vi "Turret_Manual_Aim.vi"   [LabVIEW 2011]
uses:
  StateMachineType.ctl
  Robot Global Data.vi
types:
  T1 = typedef "StateMachineType.ctl" = enum16{"Init", "Idle", "Start", "Do", "Stop"}
  T2 = typedef "WPI_MotorControlDeviceRef.ctl" = cluster{"DeviceStatus":errorcluster, "Type":enum16{"PWM", "CAN"}, "PWM":cluster{"Digital Module":T3, "PWM Channel":T4, "DeadBand":T5}, "CAN":cluster{"Device Number":u8, "Control Mode":T6, "Semaphore":T7, "Max Vout":dbl}, "Invert":bool, "TransformRef":T8, "InvTransformRef":T8}
  T3 = typedef "FPGA_TypedefDigitalModule.ctl" = enum16{"Digital Module 1", "Digital Module 2"}
  T4 = typedef "FPGA_DIOPWMChannel.ctl" = enum8{"PWM 1", "PWM 2", "PWM 3", "PWM 4", "PWM 5", "PWM 6", "PWM 7", "PWM 8", "PWM 9", "PWM 10", "Invalid"}
  T5 = typedef "WPI_PWMDeadband.ctl" = cluster{"Name":string, "maxPositivePwm":i32, "minPositivePwm":i32, "centerPwm":i32, "maxNegativePwm":i32, "minNegativePwm":i32, "angularRange":u16}
  T6 = typedef "WPI_CANJaguar_ControlMode.ctl" = enum8{"Percent VBus", "Current", "Speed", "Position", "Voltage"}
  T7 = typedef "Semaphore RefNum" = refnum<k1>
  T8 = typedef "WPI_PWMTransform_ConPane.ctl" = refnum<vi>
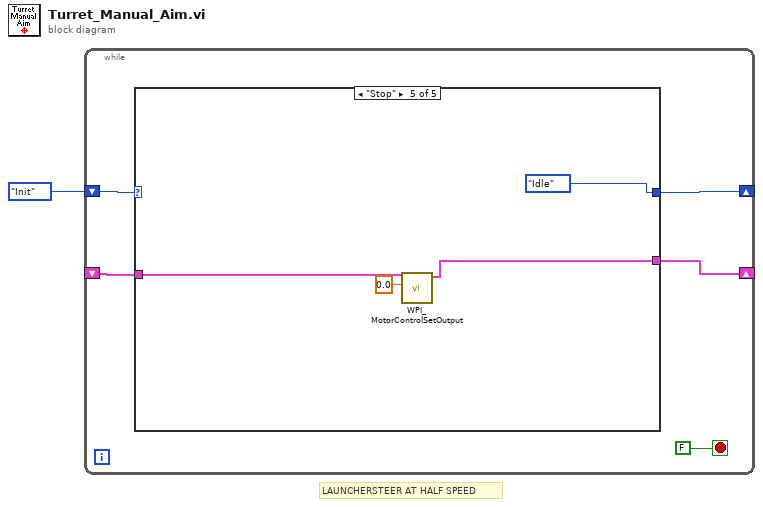
[diagram p0: block diagram]
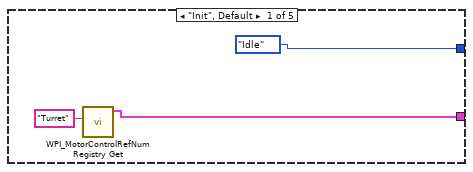
[diagram p2: hidden frame]
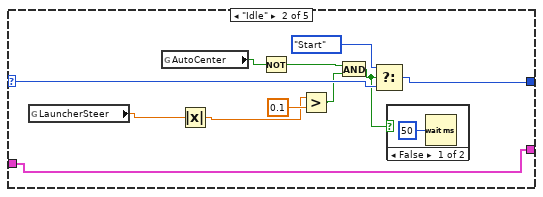
[diagram p3: hidden frame]
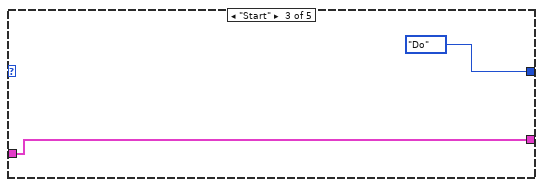
[diagram p5: hidden frame]
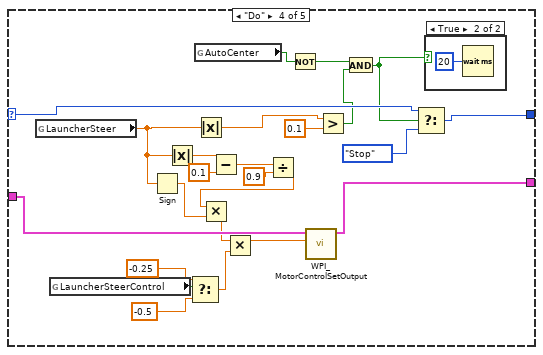
[diagram p6: hidden frame]
diagram:
  # "LAUNCHERSTEER AT HALF SPEED"
  n1 = while {
    shift-right: [w4] -> _
    shift-left: StateMachineType."Init" -> [w5]
    shift-right: [w3] -> _
    shift-left: _ -> [w2]
    stop <- FALSE stop-if-true
    n2 = case shown="\"Stop\"" w5 {
      selector: w5 -> [_ w19 _ w44 _]
      tunnel: [StateMachineType."Idle" ("Enum") w18 StateMachineType."Do" ("Enum") w45 StateMachineType."Idle" ("Enum")] -> w4
      tunnel: [w7 w16 w23 w41 w50] -> w3
      tunnel: w2 -> [_ w16 w23 w42 w51]
      frame "Init", Default {
        n3 = call <vilib>:"WPI_MotorControlRefNum Registry Get.vi"("refnum name"="Turret") -> ("MotorControlDevRef"=w7:T2)  [unwired: 9 in, 1 out]
      }
      frame "Idle" {
        n4 = global read "Robot Global Data.vi" "LauncherSteer"() -> (w15:dbl)
        n5 = global read "Robot Global Data.vi" "AutoCenter"() -> (w13:bool)
        n6 = Absolute Value(x=w15) -> (abs(x)=w14:dbl)
        n7 = Not(x=w13) -> (.not. x?=w11:bool)
        n8 = Greater?(x=w14, y=0.1) -> (0:w12:bool)
        n9 = And(x=w11, y=w12) -> (x .and. y?=w10:bool)
        n10 = Select(t=StateMachineType."Start" ("Enum"), s=w10, f=w19) -> (s? t:f=w18:T1)
        n11 = case shown="False" w10 {
          frame False {
            n12 = Wait (ms)(milliseconds to wait=u32 50) -> ()  [unwired: 1 out]
          }
          frame True {
          }
        }
      }
      frame "Start" {
      }
      frame "Do" {
        n13 = global read "Robot Global Data.vi" "LauncherSteer"() -> (w27:dbl)
        n14 = global read "Robot Global Data.vi" "LauncherSteerControl"() -> (w35:bool)
        n15 = Sign(1:w27) -> (0:w26:dbl)
        n16 = Absolute Value(x=w27) -> (abs(x)=w31:dbl)
        n17 = Select(t=-0.25 ("y"), s=w35, f=-0.5 ("y")) -> (s? t:f=w32:dbl)
        n18 = global read "Robot Global Data.vi" "AutoCenter"() -> (w39:bool)
        n19 = Absolute Value(x=w27) -> (abs(x)=w43:dbl)
        n20 = Subtract(x=w31, y=0.1) -> (x-y=w30:dbl)
        n21 = Divide(x=w30, y=0.9) -> (x/y=w25:dbl)
        n22 = Multiply(x=w25, y=w26) -> (x*y=w24:dbl)
        n23 = Multiply(x=w24, y=w32) -> (x*y=w40:dbl)
        n24 = Not(x=w39) -> (.not. x?=w36:bool)
        n25 = call <vilib>:"WPI_MotorControlSetOutput.vi"("Output"=w40, "MotorControlDevRef"=w42) -> ("MotorControlDevRef"=w41:T2)  [unwired: 8 in, 1 out]
        n26 = Greater?(x=w43, y=0.1) -> (0:w38:bool)
        n27 = And(x=w36, y=w38) -> (x .and. y?=w37:bool)
        n28 = Select(t=w44, s=w37, f=StateMachineType."Stop" ("Enum")) -> (s? t:f=w45:T1)
        n29 = case shown="True" w37 {
          frame False {
          }
          frame True {
            n30 = Wait (ms)(milliseconds to wait=u32 20) -> ()  [unwired: 1 out]
          }
        }
      }
      frame "Stop" {
        n31 = call <vilib>:"WPI_MotorControlSetOutput.vi"("Output"=0.0, "MotorControlDevRef"=w51) -> ("MotorControlDevRef"=w50:T2)  [unwired: 8 in, 1 out]
      }
    }
  }
